vi "control6acater01.vi"() -> ()   [LabVIEW 2018]
uses:
  <vilib>/Platform/TimedLoop/XDataNode/timing_clust.ctl
  <vilib>/Platform/TimedLoop/XDataNode/nitl_modes.ctl
  <vilib>/Platform/TimedLoop/XDataNode/wakeup.ctl
  <vilib>/rvi/Emulation/niFpgaSctlEmulationGetInTimedLoop.vi
  <vilib>/rvi/Emulation/niFpgaEmulationReportErrorSimple.vi
  <vilib>/rvi/Emulation/niFpgaGetClockAttributes.vi
  <vilib>/rvi/Emulation/niFpgaCriticalErrorInLSC.vi
  <vilib>/rvi/eio/common/nirviEmuTemplateMethod_errors.vi
  <vilib>/Platform/TimedLoop/XDataNode/XDataNode.xnode
  <vilib>/eio/EIONode/EIONode.xnode
  <vilib>/Platform/TimedLoop/XDataNode/XDNodeRunTimeDep.lvlib
panel:
  in  "Period (Ticks)":u32
  in  "Duty Cycle 6":fxp<+,32,0>
  in  "Duty Cycle 5":fxp<+,32,0>
  in  "Duty Cycle 4":fxp<+,32,0>
  in  "Duty Cycle 3":fxp<+,32,0>
  in  "Duty Cycle 2":fxp<+,32,0>
  in  "Duty Cycle":fxp<+,32,0>
  in  "stop":bool
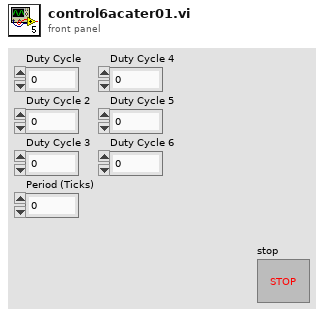
[diagram p1: front panel]
types:
  T1 = typedef "XDNodeRunTimeDep.lvlib/timing_clust.ctl" = cluster{"Expected End [f-1]":u64, "Actual End [f-1]":u64, "Finished Late? [f-1]":bool, "Expected End [i-1]":u64, "Actual End [i-1]":u64, "Finished Late? [i-1]":bool, "Expected Start [i]":u64, "Actual Start [i]":u64, "Expected Start [f]":u64, "Actual Start [f]":u64, "Source Name":string, "Structure Name":string, "Period":i64, "Deadline":i64, "Offset":i64, "Start":i64, "Priority":i32, "Timeout":i32, "Mode":T2, "Wakeup Reason":T3, "Error":errorcluster, "Source Type":string, "Secondary Source Type":string, "Global End Time":u64, "Global Start Time":u64, "Frame Duration":u64, "Iteration Duration":u64, "Assigned CPU":i32, "I/O Scan Engine Mode":u32}
  T2 = typedef "XDNodeRunTimeDep.lvlib/nitl_modes.ctl" = enum32{"No Change", "Process missed periods, maintain original phase", "Discard missed periods, maintain original phase", "Process missed periods, ignore original phase", "Discard missed periods, ignore original phase"}
  T3 = typedef "XDNodeRunTimeDep.lvlib/wakeup.ctl" = enum32{"Normal", "Aborted", "Asynchronous wakeup", "Timing source error", "Timed loop error", "Timeout"}
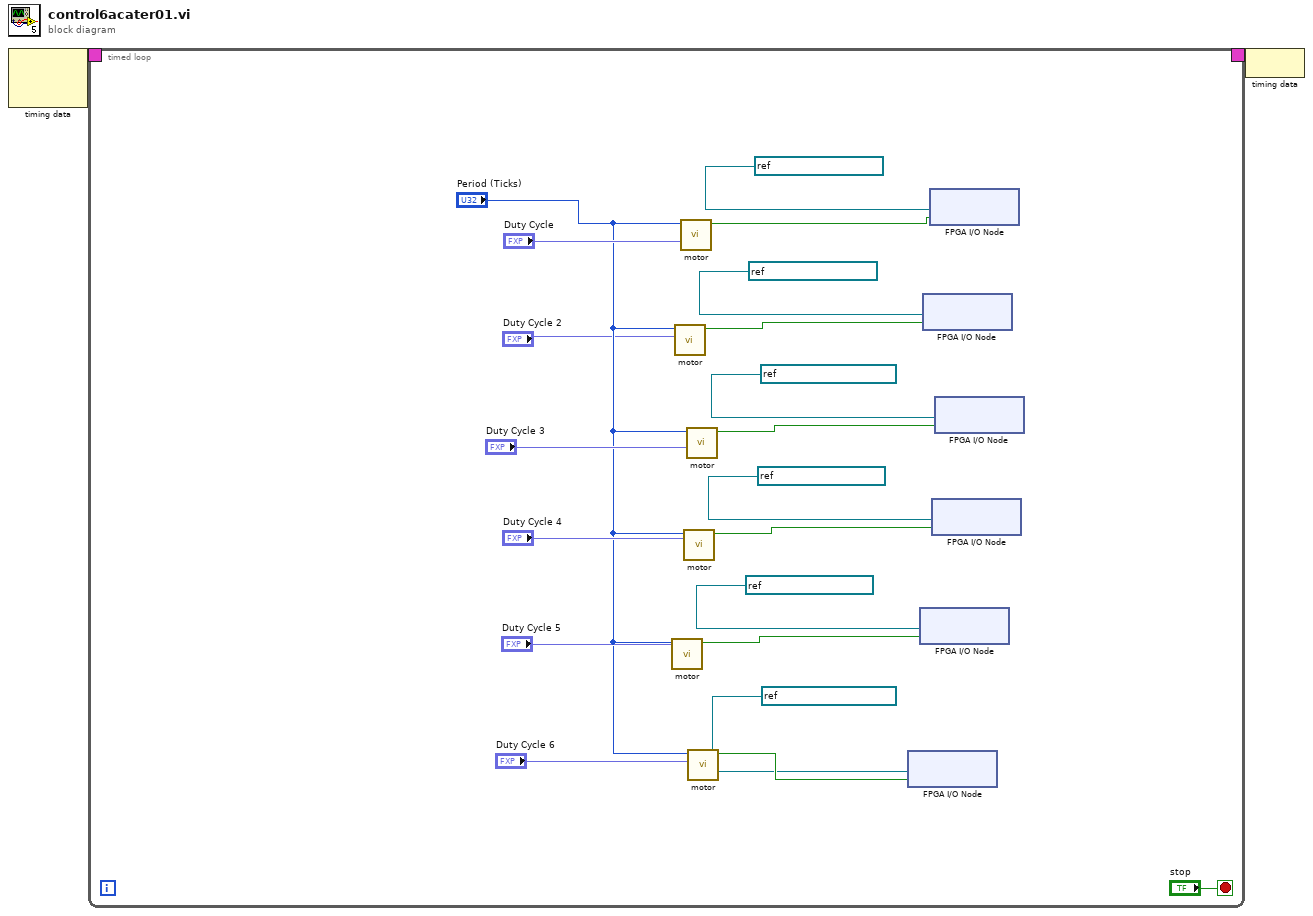
[diagram p0: block diagram]
diagram:
  n1 = node-c288() -> (w2:T1)  [unwired: 2 in]
  n2 = timed-loop {
    timing: w2 -> [_]
    timing-out: [_] -> w1
    stop <- "stop" stop-if-true
    n3 = call "motor.vi"("Duty Cycle"="Duty Cycle 5", "Period (Ticks)"="Period (Ticks)") -> ("PWM Out"=w15:bool)  [unwired: 8 in, 1 out]
    n4 = call "motor.vi"("Duty Cycle"="Duty Cycle 2", "Period (Ticks)"="Period (Ticks)") -> ("PWM Out"=w21:bool)  [unwired: 8 in, 1 out]
    n5 = call "motor.vi"("Duty Cycle"="Duty Cycle", "Period (Ticks)"="Period (Ticks)") -> ("PWM Out"=w11:bool)  [unwired: 8 in, 1 out]
    n6 = call "motor.vi"("Duty Cycle"="Duty Cycle 4", "Period (Ticks)"="Period (Ticks)") -> ("PWM Out"=w17:bool)  [unwired: 8 in, 1 out]
    n7 = call "motor.vi"("Duty Cycle"="Duty Cycle 3", "Period (Ticks)"="Period (Ticks)") -> ("PWM Out"=w19:bool)  [unwired: 8 in, 1 out]
    n8 = call "motor.vi"("Duty Cycle"="Duty Cycle 6", "Period (Ticks)"="Period (Ticks)") -> ("PWM Out"=w13:bool)  [unwired: 8 in, 1 out]
    n9 = xnode "FPGA I/O Node"("I/O Item"=w13, "FPGA I/O In"=refnum<k21> "ConnectorB/DIO10") -> ()  [unwired: 1 out]
    n10 = xnode "FPGA I/O Node"("I/O Item"=w15, "FPGA I/O In"=refnum<k21> "ConnectorB/DIO9") -> ()  [unwired: 1 out]
    n11 = xnode "FPGA I/O Node"("I/O Item"=w21, "FPGA I/O In"=refnum<k21> "ConnectorA/DIO9") -> ()  [unwired: 1 out]
    n12 = xnode "FPGA I/O Node"("I/O Item"=w11, "FPGA I/O In"=refnum<k21> "ConnectorA/DIO8") -> ()  [unwired: 1 out]
    n13 = xnode "FPGA I/O Node"("I/O Item"=w17, "FPGA I/O In"=refnum<k21> "ConnectorB/DIO8") -> ()  [unwired: 1 out]
    n14 = xnode "FPGA I/O Node"("I/O Item"=w19, "FPGA I/O In"=refnum<k21> "ConnectorA/DIO10") -> ()  [unwired: 1 out]
  }
  n15 = node-c288(w1) -> ()
